vi "Fetch Measurement (Harmonics).vi"(6 "Timeout (10000 ms)":i32=10000 min=1, 8 "error in (no error)":errorcluster, 9 "Number of Item (15)":i32=15 min=1 max=64, 10 "Measure Item (1: Plural)":i32(ring)=1 items=["One", "Plural"], 11 "VISA resource name":refnum<visa-resource-name>) -> (0 "error out":errorcluster, 1 "Measurement":dbl[][](array[numeric]), 2 "Function":string[](array[string]), 3 "VISA resource name out":refnum<visa-resource-name>)   [LabVIEW 2021, in "Yokogawa WT1800 Series.lvlib"]
doc: "Queries the harmonic measurement numeric list data."
uses:
  <instrlib>/Yokogawa WT1800 Series/Yokogawa WT1800 Series.lvlib
  <instrlib>/Yokogawa WT1800 Series/Private/Measurement Data Convert (Harmonics).vi
panel:
  # "Total        DC            1             2              3             4"
  # "ms"
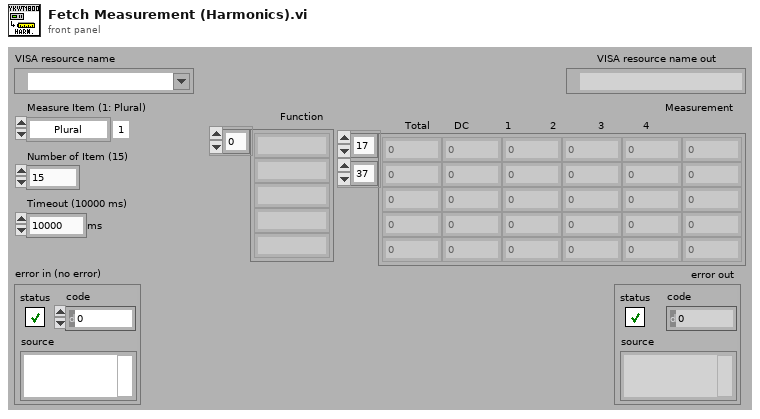
[diagram p1: front panel]
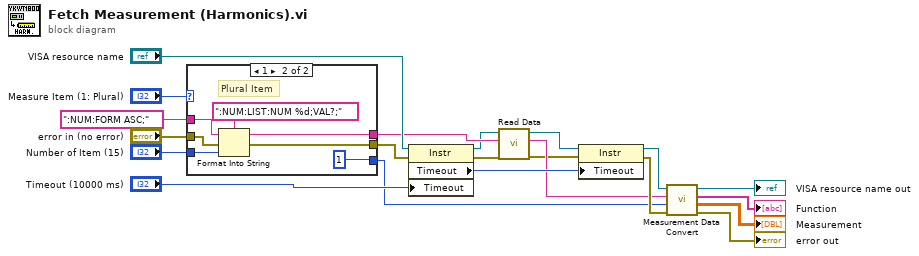
[diagram p0: block diagram]
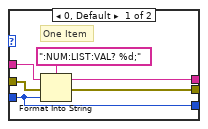
[diagram p2: hidden frame]
diagram:
  n1 = case shown="1" "Measure Item (1: Plural)" {
    tunnel: ":NUM:FORM ASC;" ("形式文字列") -> [w26 w33]
    tunnel: "Number of Item (15)" -> [w22 w32]
    tunnel: "error in (no error)" -> [w25 w31]
    tunnel: [w24 w30] -> w3
    tunnel: [w23 w29] -> w16
    tunnel: [w22 1] -> w11
    frame 0, Default {
      # "One Item"
      n2 = Format Into String(format string=":NUM:LIST:VAL? %d;" ("形式文字列"), initial string=w26, error in=w25, w22) -> (resulting string=w24:string, error out=w23:errorcluster)
    }
    frame 1 {
      # "Plural Item"
      n3 = Format Into String(format string=":NUM:LIST:NUM %d;VAL?;" ("形式文字列"), initial string=w33, error in=w31, w32) -> (resulting string=w30:string, error out=w29:errorcluster)
    }
  }
  n4 = property on="プロパティノード" class="Instr"(reference="VISA resource name", error in=w16, "Timeout"="Timeout (10000 ms)") -> (reference out=w1:refnum<visa-resource-name>, error out=w2:errorcluster, "Timeout"=w15:u32)
  n5 = call <instrlib>:"Read Data.vi"("error in (no error)"=w2, "Send Command (Empty)"=w3, "VISA resource name"=w1) -> ("error out"=w4:errorcluster, "Read Data"=w5:string, "VISA resource name out"=w6:refnum<visa-resource-name>)  [unwired: 5 in, 1 out]
  n6 = property on="プロパティノード" class="Instr"(reference=w6, error in=w4, "Timeout"=w15) -> (reference out=w13:refnum<visa-resource-name>, error out=w12:errorcluster)
  n7 = call-poly <instrlib>:"Measurement Data Convert.vi"("error in (no error)"=w12, "Item Number Offset (1)"=w11, "Measurement Data (Empty)"=w5, "VISA resource name"=w13) -> ("error out"=→"error out":errorcluster, "Measurement"=→"Measurement":dbl[][], "Function"=→"Function":string[], "VISA resource name out"=→"VISA resource name out":refnum<visa-resource-name>)  [unwired: 4 in]
